vi "Write DelayLine.vi"(8 "error in (no error)":errorcluster, 10 "DelayLine.lvclass":refnum<class "DelayLine.lvclass">, 11 "Control in":refnum<class "Control-Server.lvclass">) -> (0 "error out":errorcluster, 3 "Control out":refnum<class "Control-Server.lvclass">)   [LabVIEW 2015, in "Control-Server.lvclass"]
uses:
  Control-Server.lvclass
  Delay Line/DelayLine.lvclass
  Control-Server.lvclass/Control-Server.ctl
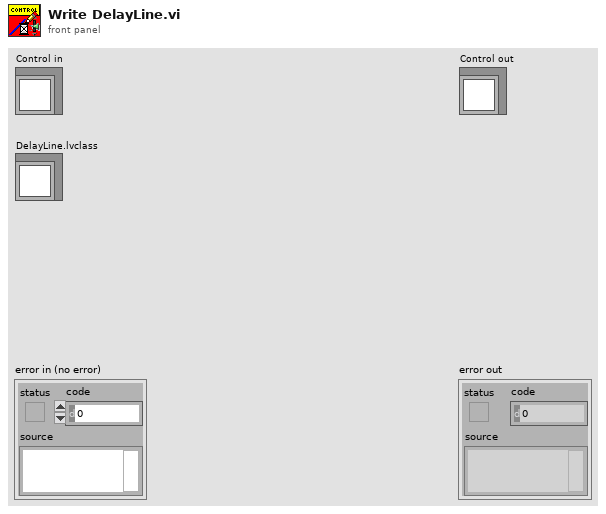
[diagram p1: front panel]
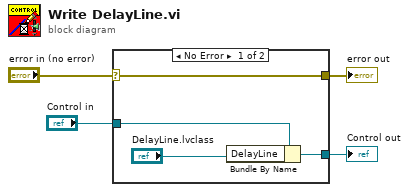
[diagram p0: block diagram]
diagram:
  n1 = case shown="No Error" "error in (no error)" {
    selector: "error in (no error)" -> [w6 w9]
    tunnel: [w6 w9] -> w3
    tunnel: [w7 w10] -> w1
    tunnel: "Control in" -> [w8 w10]
    frame No Error {
      n2 = Bundle By Name(cluster=w8, "DelayLine"="DelayLine.lvclass") -> (w7:refnum<class "Control-Server.lvclass">)
    }
    frame Error {
    }
  }
  "error out" <- w3
  "Control out" <- w1
